vi "TestifTouching.vi"(0 "Piece Array":i16[][](array[numeric]), 5 "board array":i16[][](array[numeric])) -> (6 "Lost":bool, 7 "min Distance":i16, 8 "Touching":bool)   [LabVIEW 2019]
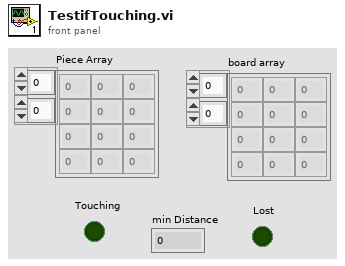
[diagram p1: front panel]
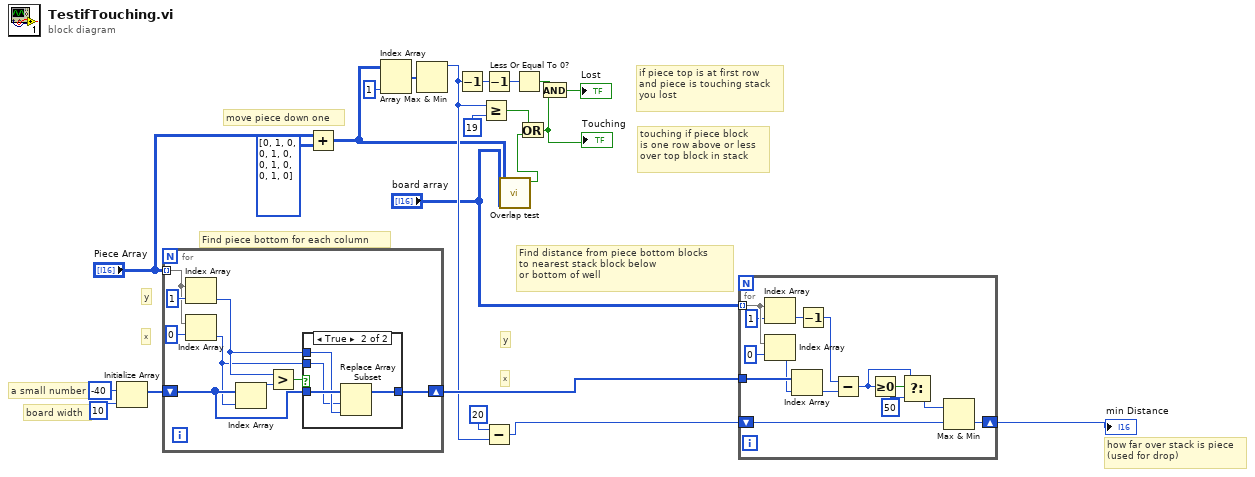
[diagram p0: block diagram]
diagram:
  # "move piece down one"
  # "a small number"
  # "how far over stack is piece\n(used for drop)"
  # "touching if piece block\nis one row above or less \nover top block in stack"
  # "if piece top is at first row\nand piece is touching stack\nyou lost"
  # "Find distance from piece bottom blocks \nto nearest stack block below\nor bottom of well"
  # "x"
  # "y"
  # "x"
  # "y"
  # "Find piece bottom for each column"
  # "board width"
  n1 = Initialize Array(i16 -40, 10) -> (w20:i16[])
  n2 = for {
    tunnel: "Piece Array" -> [w29] mode=indexing
    shift-right: [w26] -> w6
    shift-left: w20 -> [w25]
    n3 = Index Array(array=w29, index=1) -> (element=w24:i16)
    n4 = Index Array(array=w29, index=0) -> (element=w23:i16)
    n5 = Index Array(array=w25, index=w23) -> (element=w28:i16)
    n6 = Greater?(x=w24, y=w28) -> (0:w27:bool)
    n7 = case shown="True" w27 {
      tunnel: [w32 w36] -> w26
      tunnel: w25 -> [w32 w35]
      tunnel: w24 -> [_ w34]
      tunnel: w23 -> [_ w33]
      frame False {
      }
      frame True {
        n8 = Replace Array Subset(array=w35, new element=w34, index=w33) -> (w36:i16[])
      }
    }
  }
  n9 = Add(x="Piece Array", y=i32[][] [[0, 1, 0], [0, 1, 0], [0, 1, 0], [0, 1, 0]]) -> (x+y=w3:i32[][])
  n10 = Index Array(array=w3, index (col)=1) -> (element=w15:i32[])  [unwired: 1 in]
  n11 = Array Max & Min(array=w15) -> (max value=w5:i32)  [unwired: 3 out]
  n12 = Decrement(x=w5) -> (x-1=w14:i32)
  n13 = Greater Or Equal?(x=w5, y=19) -> (x >= y?=w8:bool)
  n14 = Decrement(x=w14) -> (x-1=w4:i32)
  n15 = Subtract(x=20, y=w5) -> (x-y=w10:i32)
  n16 = call "Overlap test.vi"("Stack Array"="board array", "Piece Array"=w3) -> ("Interference"=w1:bool)  [unwired: 9 in]
  n17 = Less Or Equal To 0?(x=w4) -> (x <= 0?=w13:bool)
  n18 = Or(x=w8, y=w1) -> (x .or. y?=w7:bool)
  "Touching" <- w7
  n19 = And(x=w13, y=w7) -> (x .and. y?=→"Lost":bool)
  n20 = for {
    tunnel: "board array" -> [w50] mode=indexing
    tunnel: w6 -> [w47]
    shift-right: [w44] -> w19
    shift-left: w10 -> [w43]
    n21 = Index Array(array=w50, index=1) -> (element=w45:i16)
    n22 = Index Array(array=w50, index=0) -> (element=w46:i16)
    n23 = Index Array(array=w47, index=w46) -> (element=w41:i16)
    n24 = Decrement(x=w45) -> (x-1=w42:i16)
    n25 = Subtract(x=w42, y=w41) -> (x-y=w37:i16)
    n26 = Greater Or Equal To 0?(x=w37) -> (x >= 0?=w40:bool)
    n27 = Select(t=w37, s=w40, f=50) -> (s? t:f=w38:i32)
    n28 = Max & Min(x=w38, y=w43) -> (min(x,y)=w44:i32)  [unwired: 1 out]
  }
  "min Distance" <- w19
